vi "Allan Variance Chart O.vi"(8 "error in (no error)":errorcluster, 9 "nArray":i32[](array[numeric]) min=1 step=1, 11 "inputdata":dbl[](array[numeric])) -> (0 "error out":errorcluster, 2 "Allan Deviation":dbl[](array[numeric]), 3 "Allan Variance":dbl[](array[numeric]))   [LabVIEW 2021, in "IMU Processing.lvlib" / "ErrorModellingLibrary.lvlib"]
doc: "extern \"C\" ERRORMODELLIBRARY_API void allanVarianceChartO(float* inputdata, float* outputdata, int N);\n\nextern \"C\" ERRORMODELLIBRARY_API void allanVarianceChartO(float* inputdata, float* outputdata, int N, int* nArray, int nLength);"
uses:
  ErrorModellingLibrary.lvlib
  ErrorModellingLibrary.dll
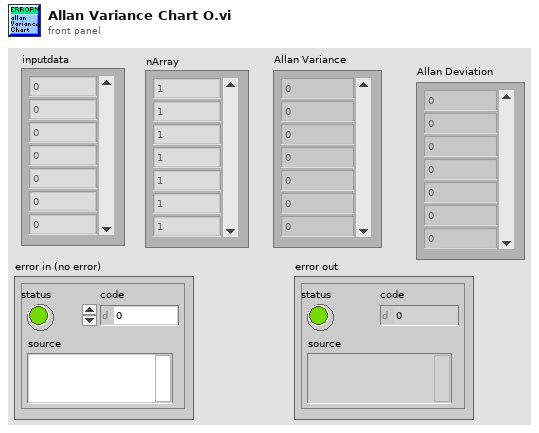
[diagram p1: front panel]
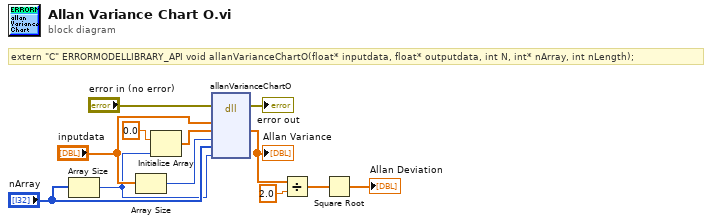
[diagram p0: block diagram]
diagram:
  # "extern \"C\" ERRORMODELLIBRARY_API void allanVarianceChartO(float* inputdata, float* outputdata, int N, int* nArray, int nLength);"
  n1 = Array Size(array="nArray") -> (size(s)=w5:i32)
  n2 = Array Size(array="inputdata") -> (size(s)=w7:i32)
  n3 = Initialize Array(sgl 0.0 ("element"), w5) -> (w12:sgl[])
  n4 = dll-call lib="E:/Documents/Thesis/IMU-ICM-20948/Computer/Labview/Thesis/IMU/Processing/ErrorModellingLibrary/ErrorModellingLibrary.*" fn="allanVarianceChartO"(error in="error in (no error)", "inputdata"="inputdata", "outputdata"=w12, "N"=w7, "nArray"="nArray", "nLength"=w5) -> (error out=→"error out":errorcluster, "outputdata"=w4:sgl[])  [unwired: 7 in, 1 out]
  "Allan Variance" <- w4
  n5 = Divide(x=w4, y=sgl 2.0) -> (x/y=w2:sgl[])
  n6 = Square Root(x=w2) -> (sqrt(x)=→"Allan Deviation":sgl[])
